vi "ModuleManager.vi"(10 "Parameters":variant, 11 "Process":refnum<class "Process.lvclass">) -> ()   [LabVIEW 2018, in "Vires VTD Engine.lvlib"]
uses:
  Vires VTD Engine.lvlib
  <vilib>/NI/NIVS Inline Async API/_VS Inline Async API/Process/Process.lvclass
  Shared/Compiled.Settings.ctl
  System Explorer/RDB Data.ctl
  RDB/RDB Object.ctl
  RDB/RDB Player Object.ctl
  Shared/Network Settings.ctl
  Shared/Protocol.ctl
  Shared/SensorInfos.ctl
  Shared/SensorInfo.ctl
  Shared/Sensor Name.ctl
  MM/MM Data.ctl
  MM/MM Objects.ctl
  MM/MM Object.ctl
  <vilib>/NI/NIVS Inline Async API/_VS Inline Async API/Process/Process.lvclass/Process.ctl
  <vilib>/NI/NIVS Inline Async API/_Data Access Engine/Access Type Classes/Write/Write.lvclass/Write.ctl
  <vilib>/NI/NIVS Inline Async API/_Data Access Engine/Data Access Engine/Methods/Write.Data.vi
  <vilib>/NI/NIVS Inline Async API/_VS Inline Async API/Process/Data Member Access/Read Data Access.vi
  <vilib>/NI/NIVS Inline Async API/_VS Inline Async API/Error Handling Process/SubVIs/Error.ConvertArray.vi
  <vilib>/NI/NIVS Inline Async API/_Data Access Engine/Access Type Classes/Write/Write.ProcessData.vi
  <vilib>/NI/NIVS Inline Async API/_Data Access Engine/Access Type Classes/Write/Write.Buffer.vi
  <vilib>/NI/NIVS Inline Async API/_Data Access Engine/Access Type Classes/Write/Write.Commit.vi
  <vilib>/NI/NIVS Inline Async API/_Data Access Engine/Data Access Engine/Methods/Write.Lookup.vi
  <vilib>/NI/NIVS Inline Async API/_Data Access Engine/Data Access Engine/Data Access Engine.lvclass
  Shared/Vires VTD Shared.lvlib
  RDB/RDB.lvlib
  MM/MM.lvlib
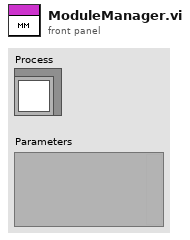
[diagram p1: front panel]
types:
  T1 = typedef "Vires VTD Shared.lvlib/Compiled.Settings.ctl" = cluster{"Name":string, "RDB Data Receive ":T2, "RDB Data Sent":T2, "vclient":path, "Network Settings":T5, "SensorInfos":T7, "mmanager":path, "Scenario Paths":string[], "Custom SCP Commands":string[]}
  T2 = typedef "Vires VTD Shared.lvlib/RDB Data.ctl" = T3[]
  T3 = typedef "RDB.lvlib/RDB Object.ctl" = cluster{"pkID":i32, "RDB Player Objects":T4[]}
  T4 = typedef "RDB.lvlib/RDB Player Object.ctl" = cluster{"PlayerID":i32, "Signals":string[], "WheelID":i32}
  T5 = typedef "Vires VTD Shared.lvlib/Network Settings.ctl" = cluster{"IP adress":string, "RDB":cluster{"Protocol":T6, "Tx Port":u16, "Rx Port":u16, "Buffer Size":i32, "Timeout":u16}, "SCP":cluster{"Protocol":T6, "Tx Port":u16, "Rx Port":u16, "Buffer Size":i32, "Timeout":u16}}
  T6 = typedef "Vires VTD Shared.lvlib/Protocol.ctl" = enum16{"UDP", "TCP"}
  T7 = typedef "Vires VTD Shared.lvlib/SensorInfos.ctl" = T8[]
  T8 = typedef "Vires VTD Shared.lvlib/SensorInfo.ctl" = cluster{"Sensor Name":T9, "Protocol":T6, "Network port":i32, "# Culled Objects":i32, "PlayerID":u8, "MM Data":T10}
  T9 = typedef "Vires VTD Shared.lvlib/Sensor Name.ctl" = string
  T10 = typedef "Vires VTD Shared.lvlib/MM Data.ctl" = T11[]
  T11 = typedef "MM.lvlib/MM Objects.ctl" = cluster{"pkID":i32, "MM Objects":T12[]}
  T12 = typedef "MM.lvlib/MM Object.ctl" = cluster{"Object":i32, "Signals":string[]}
  T13 = typedef "Data Access Engine.lvlib/Data Access Engine.lvclass/Write.DVR.ctl" = refnum<data-value>
  T14 = typedef "MM.lvlib/Sensor Engine Data.ctl" = cluster{"TCP Network":refnum<k5>, "UDP Network":refnum<k16>, "Network port":i32, "Protocol":T6, "Sensor Name":T9, "Signal Data":dbl[], "MM Frames":T15[], "MM Culled Objects":i32[], "MM Frame Refs":refnum<k21>[], "mmanager":path}
  T15 = typedef "XNET Frame FlexRay.ctl" = cluster{"timestamp":timestamp, "payload":u8[], "slot":u16, "type":T16, "cycle count":u8, "startup?":bool, "sync?":bool, "preamble?":bool, "ch A":bool, "ch B":bool, "echo?":bool}
  T16 = typedef "XNET Frame Type FlexRay.ctl" = u8
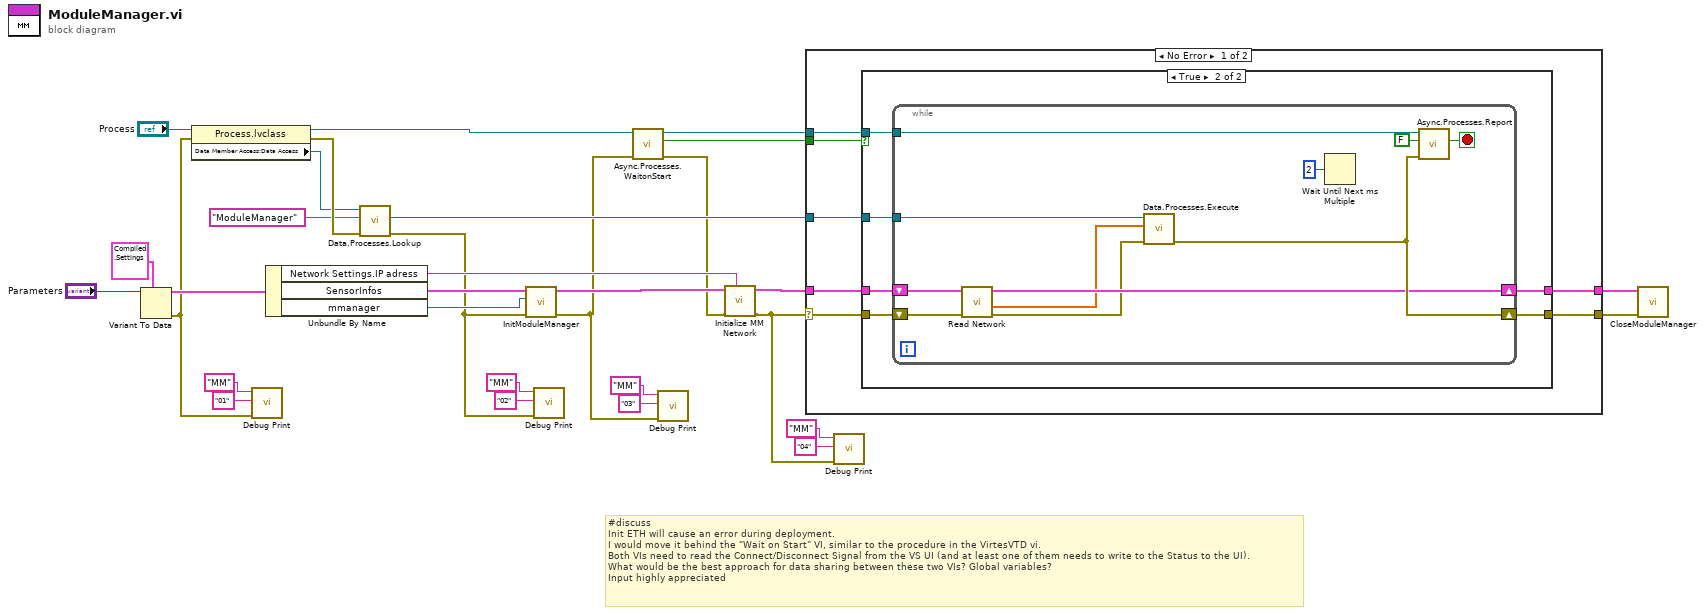
[diagram p0: block diagram]
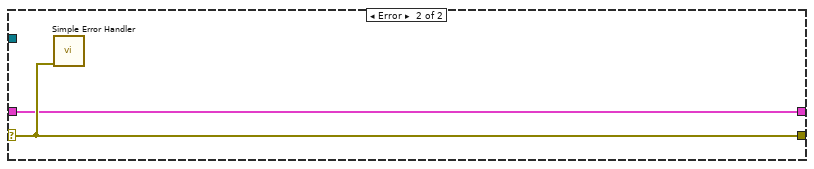
[diagram p3: hidden frame]
diagram:
  # "#discuss\nInit ETH will cause an error during deployment.\nI would move it behind the \"Wait on Start\" VI, similar to the procedure in the VirtesVTD vi.\nBoth VIs need to read the Connect/Disconnect Signal from the VS UI (and at least one of them needs to write to the Status to the UI).\nWhat would be the best approach for data sharing between these two VIs? Global variables?\nInput highly appreciated"
  n1 = Variant To Data(type=T1 {"Name"="", "RDB Data Receive "=[], "RDB Data Sent"=[], "vclient"=path "", "Network Settings"={"IP adress"="127.0.0.1", "RDB"={"Protocol"=enum."TCP", "Tx Port"=10, "Rx Port"=10, "Buffer Size"=204800, "Timeout"=10}, "SCP"={"Protocol"=enum."UDP", "Tx Port"=48190, "Rx Port"=48190, "Buffer Size"=204800, "Timeout"=10}}, "SensorInfos"=[], "mmanager"=path "", "Scenario Paths"=[], "Custom SCP Commands"=[]} ("Compiled.Settings"), Variant="Parameters") -> (data=w21:T1, error out=w11:errorcluster)  [unwired: 1 in]
  n2 = property class="Process.lvclass"(reference="Process", error in=w11) -> (reference out=w28:refnum<class "Process.lvclass">, error out=w25:errorcluster, "Data Member Access:Data Access"=w24:refnum<class "Data Access Engine.lvclass">)
  n3 = call "Debug Print.vi"("error out"=w11, "Index"="01", "Module"="MM") -> ()  [unwired: 9 in]
  n4 = Unbundle By Name(w21) -> ("Network Settings.IP adress"=w18:string, "SensorInfos"=w17:T7, "mmanager"=w14:path)
  n5 = call-poly <vilib>:"Data.Processes.Lookup.vi"("error in (no error)"=w25, "Name"="ModuleManager" ("Item Name"), "Data Access API in"=w24) -> ("error out"=w8:errorcluster, "Ref"=w22:T13)  [unwired: 5 in, 2 out]
  n6 = call "InitModuleManager.vi"("error in (no error)"=w8, "mmanager"=w14, "SensorInfos"=w17) -> ("error out (no error)"=w3:errorcluster, "Sensor Engine Datas"=w20:T14[])  [unwired: 7 in]
  n7 = call "Debug Print.vi"("error out"=w8, "Index"="02", "Module"="MM") -> ()  [unwired: 9 in]
  n8 = call <vilib>:"Async.Processes.WaitonStart.vi"("error in (no error)"=w3, "Process"=w28) -> ("error out"=w2:errorcluster, "Execute"=w31:bool, "Process out"=w30:refnum<class "Process.lvclass">)  [unwired: 7 in]
  n9 = call "Debug Print.vi"("error out"=w3, "Index"="03", "Module"="MM") -> ()  [unwired: 9 in]
  n10 = call "Initialize MM Network.vi"("Net Adress"=w18, "error in (no error)"=w2, "Sensor Engine Datas in"=w20) -> ("error out"=w1:errorcluster, "Sensor Engine Datas out"=w19:T14[])  [unwired: 7 in]
  n11 = case shown="No Error" w1 {
    selector: w1 -> [w36 w59]
    tunnel: w31 -> [w38 _]
    tunnel: w30 -> [w37 _]
    tunnel: w22 -> [w35 _]
    tunnel: [w34 w59] -> w16
    tunnel: w19 -> [w33 w58]
    tunnel: [w32 w58] -> w15
    frame No Error {
      n12 = case shown="True" w38 {
        tunnel: w36 -> [w40 w46]
        tunnel: w37 -> [_ w45]
        tunnel: w35 -> [_ w44]
        tunnel: [w40 w43] -> w34
        tunnel: w33 -> [w39 w42]
        tunnel: [w39 w41] -> w32
        frame False {
        }
        frame True {
          n13 = while {
            tunnel: w45 -> [w57]
            tunnel: w44 -> [w54]
            shift-right: [w53] -> w43
            shift-left: w46 -> [w52]
            shift-right: [w50] -> w41
            shift-left: w42 -> [w51]
            stop <- w56 stop-if-true
            n14 = call "Read Network.vi"("error in (no error)"=w52, "Sensor Engine Datas in"=w51) -> ("error out"=w49:errorcluster, "signal data"=w48:dbl[], "Sensor Engine Datas out"=w50:T14[])  [unwired: 6 in, 1 out]
            n15 = call-poly <vilib>:"Data.Processes.Execute.vi"("error in (no error)"=w49, "Values"=w48, "Ref"=w54) -> ("error out"=w53:errorcluster)  [unwired: 8 in]
            n16 = Wait Until Next ms Multiple(millisecond multiple=u32 2) -> ()  [unwired: 1 out]
            n17 = call <vilib>:"Async.Processes.Report.vi"("Error"=w53, "Stop Async on Error?"=FALSE, "Process in"=w57) -> ("Stop"=w56:bool)  [unwired: 7 in, 1 out]
          }
        }
      }
    }
    frame Error {
      n18 = call <vilib>:"Simple Error Handler.vi"("error in (no error)"=w59) -> ()  [unwired: 4 in, 5 out]
    }
  }
  n19 = call "Debug Print.vi"("error out"=w1, "Index"="04", "Module"="MM") -> ()  [unwired: 9 in]
  n20 = call "CloseModuleManager.vi"("error in (no error)"=w16, "Sensor Engine Datas in"=w15) -> ()  [unwired: 8 in, 2 out]
